vi "oa_Scaled Window (1 Channel).vi"(0 "resampled signal":cluster{"r0":dbl, "dr":dbl, "Y":dbl[]}={"r0"=0.0, "dr"=1.0, "Y"=[]} {"r0" format="%.2p"; "dr" format="%.2p"; "Y" format="%.2f"}, 1 "processing control in":T1(ring), 7 "spectrum settings":cluster{"window type":u32, "block size":i32}={"window type"=1, "block size"=400} {"block size" min=2; "window type" items=["None"=0, "Hanning"=1, "Hamming"=2, "Blackman-Harris"=3, "Exact Blackman"=4, "Blackman"=5, "Flat Top"=6, "4 Term B-Harris"=7, "7 Term B-Harris"=8, "Low Sidelobe"=9, "Gaussian"=62]}, 11 "error in":errorcluster) -> (3 "dup processing control":T1(ring), 4 "Y":dbl[][](array[numeric]) format="%.7f", 6 "new spectrum available?":bool, 8 "spectrum settings":cluster{"window type":u32, "block size":i32}={"window type"=1, "block size"=400} {"block size" min=2; "window type" items=["None"=0, "Hanning"=1, "Hamming"=2, "Blackman-Harris"=3, "Exact Blackman"=4, "Blackman"=5, "Flat Top"=6, "4 Term B-Harris"=7, "7 Term B-Harris"=8, "Low Sidelobe"=9, "Gaussian"=62]}, 15 "error out":errorcluster)   [LabVIEW 2017, in "SoundVib_Resampling.lvlib"]
uses:
  <vilib>/addons/Sound and Vibration/Order Analysis/Resample Order Tracking/SoundVib_Resampling.lvlib
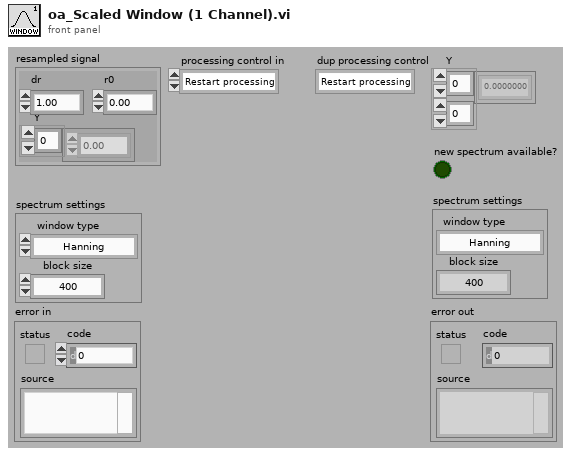
[diagram p1: front panel]
types:
  T1 = enum16{"Restart processing", "Continue processing", "Skip processing"}
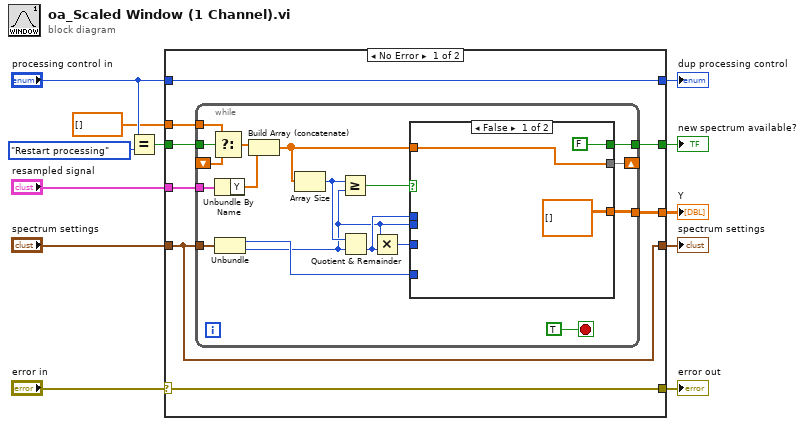
[diagram p0: block diagram]
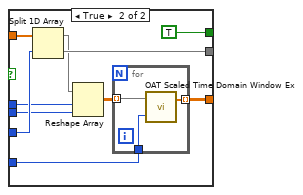
[diagram p2: hidden frame]
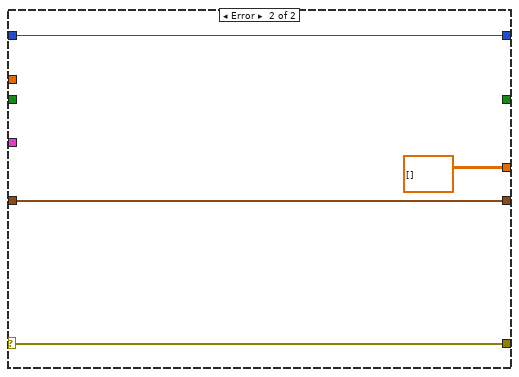
[diagram p3: hidden frame]
diagram:
  n1 = Equal?(x="processing control in", y=T1."Restart processing" ("processing control in")) -> (x = y?=w3:bool)
  n2 = case shown="No Error" "error in" {
    selector: "error in" -> [w20 w58]
    tunnel: [w20 w58] -> w11
    tunnel: "resampled signal" -> [w19 _]
    tunnel: "spectrum settings" -> [w18 w57]
    tunnel: [w18 w57] -> w8
    tunnel: [w17 dbl[][] [] ("y")] -> w7
    tunnel: "processing control in" -> [w14 w55]
    tunnel: [w14 w55] -> w6
    tunnel: w3 -> [w16 _]
    tunnel: dbl[] [] ("t") -> [w15 _]
    tunnel: [w13 _] -> w1
    frame No Error {
      n3 = while {
        tunnel: w19 -> [w37]
        shift-right: [w33] -> _
        shift-left: _ -> [w31]
        tunnel: w18 -> [w36]
        tunnel: [w28] -> w17
        tunnel: w16 -> [w32]
        tunnel: w15 -> [w30]
        tunnel: [w21] -> w13
        stop <- TRUE stop-if-true
        n4 = Select(t=w30, s=w32, f=w31) -> (s? t:f=w29:dbl[])
        n5 = Unbundle By Name(w37) -> ("Y"=w35:dbl[])
        n6 = Unbundle(w36) -> ("window type"=w27:u32, "block size"=w22:i32)
        n7 = Build Array (concatenate)(w29, w35) -> (w34:dbl[])
        n8 = Array Size(array=w34) -> (size(s)=w25:i32)
        n9 = Greater Or Equal?(x=w25, y=w22) -> (x >= y?=w26:bool)
        n10 = Quotient & Remainder(x=w25, y=w22) -> (floor(x/y)=w23:i32)  [unwired: 1 out]
        n11 = Multiply(x=w22, y=w23) -> (x*y=w24:i32)
        n12 = case shown="False" w26 {
          tunnel: w34 -> [w41 w51]
          tunnel: [w41 w49] -> w33
          tunnel: w24 -> [_ w50]
          tunnel: w23 -> [_ w47]
          tunnel: [dbl[][] [] w45] -> w28
          tunnel: w22 -> [_ w46]
          tunnel: w27 -> [_ w43]
          tunnel: [FALSE TRUE] -> w21
          frame False {
          }
          frame True {
            n13 = Split 1D Array(array=w51, index=w50) -> (first subarray=w48:dbl[], second subarray=w49:dbl[])
            n14 = Reshape Array(w48, w47, w46) -> (w44:dbl[][])
            n15 = for {
              tunnel: w44 -> [w54] mode=indexing
              tunnel: w43 -> [w53]
              tunnel: [w52] -> w45 mode=indexing
              n16 = call <vilib>:"OAT Scaled Time Domain Window Ex.vi"("window type"=w53, "X"=w54) -> ("y"=w52:dbl[])  [unwired: 1 out]
            }
          }
        }
      }
    }
    frame Error {
    }
  }
  "error out" <- w11
  "spectrum settings" <- w8
  "dup processing control" <- w6
  "Y" <- w7
  "new spectrum available?" <- w1
